vi "acquireTest.vi"() -> ()   [LabVIEW 2018]
uses:
  main/PCI8552B_32.dll
panel:
  out "字符串 2":string
  out "字符串":string
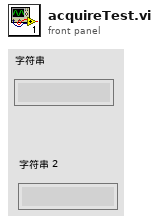
[diagram p1: front panel]
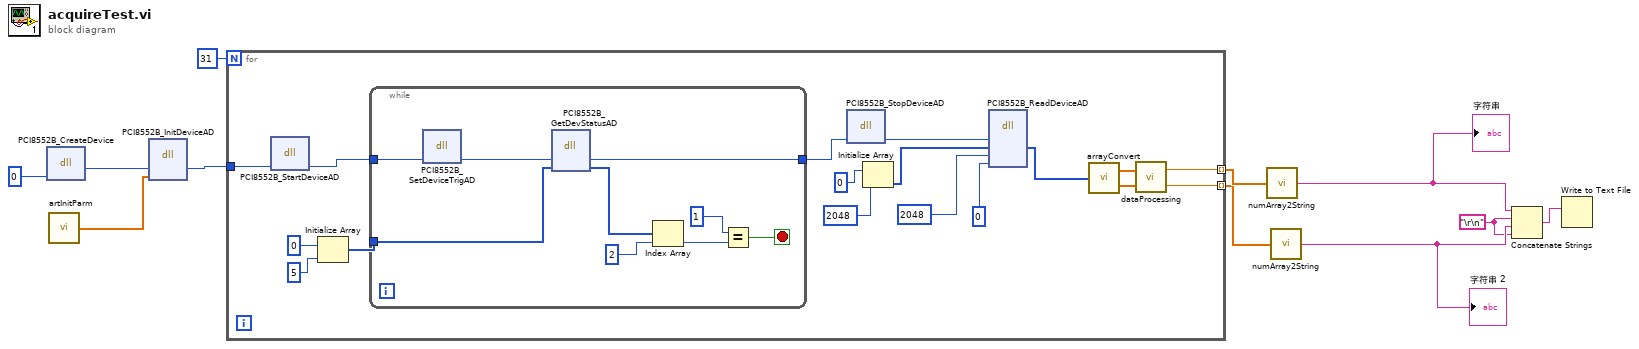
[diagram p0: block diagram]
diagram:
  w1 = "\r\n"
  n1 = dll-call lib="C:/Users/BlueMess/Desktop/Work2020/SAR Controller/SAR-Controller/main/PCI8552B_32.dll" fn="PCI8552B_CreateDevice" label="CreateDevice"("DeviceLgcID"=0) -> ("返回类型"=w10:i32)  [unwired: 4 in, 2 out]
  n2 = call "artInitParm.vi"() -> ("初始化参数"=w11:dbl[])
  n3 = dll-call lib="C:/Users/BlueMess/Desktop/Work2020/SAR Controller/SAR-Controller/main/PCI8552B_32.DLL" fn="PCI8552B_InitDeviceAD" label="InitDeviceAD"("hDevice"=w10, "pADPara"=w11) -> ("hDevice"=w7:i32)  [unwired: 5 in, 2 out]
  n4 = for {
    N: 31 -> [_]
    tunnel: w7 -> [w20]
    tunnel: [w13] -> w6 mode=indexing
    tunnel: [w12] -> w5 mode=indexing
    n5 = dll-call lib="C:/Users/BlueMess/Desktop/Work2020/SAR Controller/SAR-Controller/main/PCI8552B_32.DLL" fn="PCI8552B_StartDeviceAD" label="StartDeviceAD"("hDevice"=w20) -> ("hDevice"=w23:i32)  [unwired: 4 in, 2 out]
    n6 = Initialize Array(0, 5) -> (w21:i32[])
    n7 = while {
      tunnel: w23 -> [w32]
      tunnel: w21 -> [w37]
      tunnel: [w30] -> w22
      stop <- w29 stop-if-true
      n8 = dll-call lib="C:/Users/BlueMess/Desktop/Work2020/SAR Controller/SAR-Controller/main/PCI8552B_32.DLL" fn="PCI8552B_SetDeviceTrigAD" label="SetDeviceTrigAD"("hDevice"=w32) -> ("hDevice"=w31:i32)  [unwired: 4 in, 2 out]
      n9 = dll-call lib="C:/Users/BlueMess/Desktop/Work2020/SAR Controller/SAR-Controller/main/PCI8552B_32.DLL" fn="PCI8552B_GetDevStatusAD" label="GetDevStatusAD"("hDevice"=w31, "ADStatus"=w37) -> ("hDevice"=w30:i32, "ADStatus"=w33:i32[])  [unwired: 4 in, 2 out]
      n10 = Index Array(array=w33, index=2) -> (element=w35:i32)
      n11 = Equal?(x=1, y=w35) -> (x = y?=w29:bool)
    }
    n12 = dll-call lib="C:/Users/BlueMess/Desktop/Work2020/SAR Controller/SAR-Controller/main/PCI8552B_32.DLL" fn="PCI8552B_StopDeviceAD" label="StopDeviceAD"("hDevice"=w22) -> ("hDevice"=w17:i32)  [unwired: 4 in, 2 out]
    n13 = Initialize Array(u16 0 ("y"), 2048 ("y")) -> (w28:u16[])
    n14 = dll-call lib="C:/Users/BlueMess/Desktop/Work2020/SAR Controller/SAR-Controller/main/PCI8552B_32.DLL" fn="PCI8552B_ReadDeviceAD" label="ReadDeviceAD"("hDevice"=w17, "pADBuffer"=w28, "nReadSizeWords"=2048 ("y"), "nRetSizeWords"=u16 0 ("y")) -> ("pADBuffer"=w16:u16[])  [unwired: 7 in, 2 out]
    n15 = call "arrayConvert.vi"("输入数组"=w16) -> ("ch0"=w15:dbl[], "ch1"=w14:dbl[])
    n16 = call "dataProcessing.vi"("参考信号"=w14, "中频信号"=w15) -> ("mean_Q"=w12:dbl, "mean_I"=w13:dbl)
  }
  n17 = call "numArray2String.vi"("输入数组"=w6) -> ("输出字符串"=w3:string)
  "字符串" <- w3
  n18 = call "numArray2String.vi"("输入数组"=w5) -> ("输出字符串"=w2:string)
  "字符串 2" <- w2
  n19 = Concatenate Strings(w3, w1, w2, w1) -> (w4:string)
  n20 = Write to Text File(text=w4) -> ()  [unwired: 3 in, 3 out]
